vi "Clear All Discretes.vi"(8 "error in":errorcluster, 11 "6512 in":refnum<class "6512.lvclass">) -> (0 "error out":errorcluster, 3 "6512 out":refnum<class "6512.lvclass">)   [LabVIEW 2019, in "6512.lvlib" / "6512.lvclass"]
uses:
  Library/6512.lvclass
  builds/Instruments/DIG_IO.lvlibp/Library/DIG_IO.lvclass
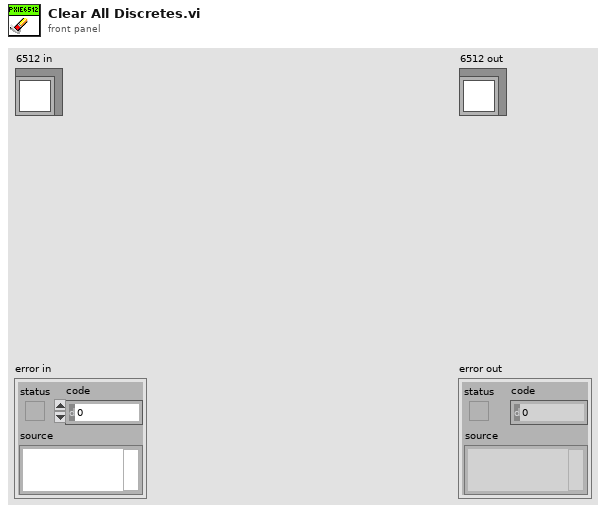
[diagram p1: front panel]
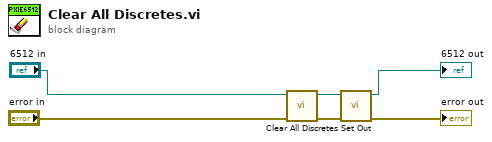
[diagram p0: block diagram]
diagram:
  n1 = call-parent "Clear All Discretes.vi"("error in"="error in", "DIG_IO in"="6512 in") -> ("error out"=w6:errorcluster, "DIG_IO out"=w5:refnum<class "6512.lvclass">)  [unwired: 8 in]
  n2 = call-dynamic "Set Out.vi"("error in"=w6, "6512 in"=w5) -> ("error out"=→"error out":errorcluster, "6512 out"=→"6512 out":refnum<class "6512.lvclass">)  [unwired: 8 in]
